vi "downloadBotSpeak.vi"() -> ()   [LabVIEW 2012]
panel:
  out "Current task":string
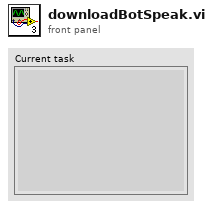
[diagram p1: front panel]
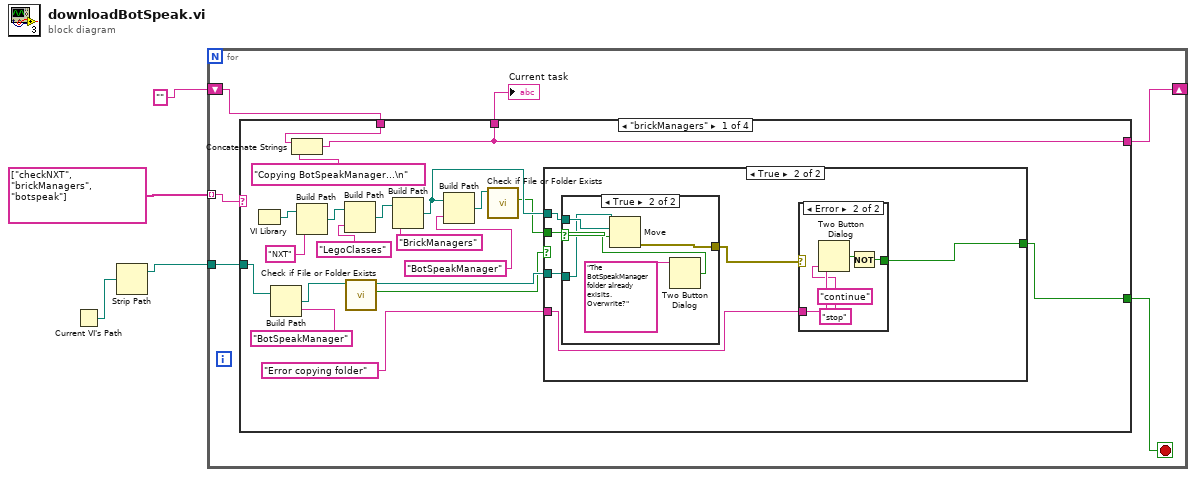
[diagram p0: block diagram]
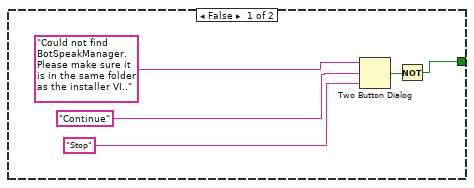
[diagram p2: hidden frame]
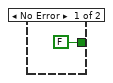
[diagram p3: hidden frame]
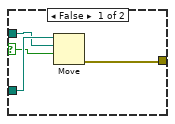
[diagram p4: hidden frame]
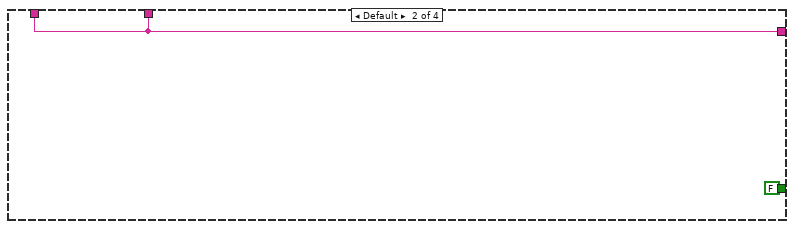
[diagram p5: hidden frame]
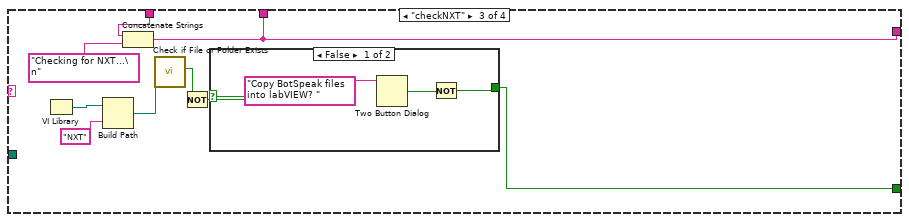
[diagram p6: hidden frame]
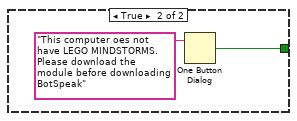
[diagram p7: hidden frame]
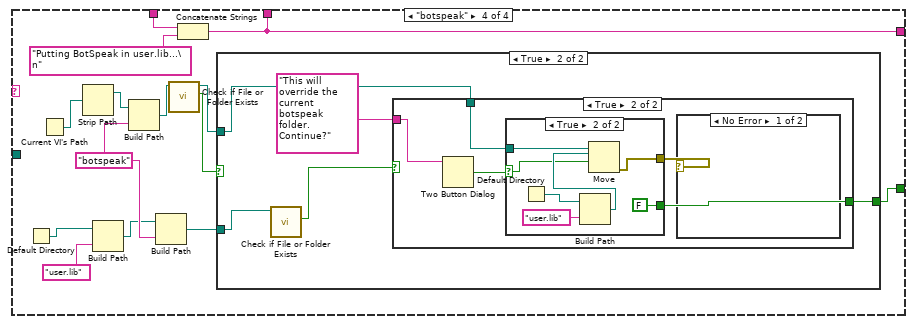
[diagram p8: hidden frame]
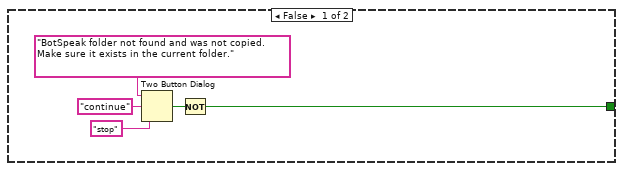
[diagram p9: hidden frame]
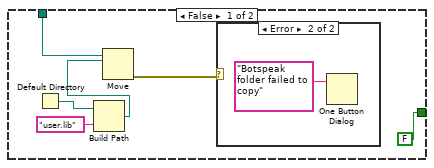
[diagram p10: hidden frame]
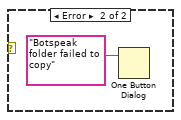
[diagram p12: hidden frame]
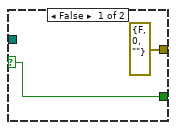
[diagram p13: hidden frame]
diagram:
  n1 = Current VI's Path() -> (path=w3:path)
  n2 = Strip Path(path=w3) -> (stripped path=w2:path)  [unwired: 1 out]
  n3 = for {
    tunnel: string[] ["checkNXT", "brickManagers", "botspeak"] -> [w10] mode=indexing
    tunnel: w2 -> [w9]
    shift-right: [w8] -> _
    shift-left: "" -> [w6]
    stop <- w7 stop-if-true
    n4 = case shown="\"brickManagers\"" w10 {
      tunnel: w9 -> [w25 _ _ _]
      tunnel: w6 -> [w15 w57 w62 w86]
      tunnel: [w11 w57 w59 w73] -> w8
      tunnel: [w12 FALSE ("T button?") w60 w79] -> w7
      tunnel: [w11 w57 w59 w73] -> w5
      frame "brickManagers" {
        n5 = VI Library() -> (path=w30:path)
        n6 = Build Path(base path=w25, name or relative path="BotSpeakManager") -> (appended path=w17:path)
        n7 = Concatenate Strings(w15, "Copying BotSpeakManager...\n" ("string")) -> (w11:string)
        n8 = Build Path(base path=w30, name or relative path="NXT") -> (appended path=w23:path)
        n9 = Build Path(base path=w23, name or relative path="LegoClasses") -> (appended path=w29:path)
        n10 = call <vilib>:"Check if File or Folder Exists.vi"("path"=w17) -> ("file or folder exists?"=w16:bool, "dup path"=w18:path)  [unwired: 8 in, 1 out]
        n11 = Build Path(base path=w29, name or relative path="BrickManagers") -> (appended path=w22:path)
        n12 = Build Path(base path=w22, name or relative path="BotSpeakManager") -> (appended path=w20:path)
        n13 = call <vilib>:"Check if File or Folder Exists.vi"("path"=w20) -> ("file or folder exists?"=w19:bool)  [unwired: 8 in, 2 out]
        n14 = case shown="True" w16 {
          tunnel: w22 -> [_ w41]
          tunnel: w19 -> [_ w40]
          tunnel: w18 -> [_ w39]
          tunnel: "Error copying folder" -> [_ w37]
          tunnel: [w31 w36] -> w12
          frame False {
            n15 = Two Button Dialog(message="Could not find BotSpeakManager. Please make sure it is in the same folder as the installer VI..", 1:"Stop" ("F button name (\"Cancel\")"), 2:"Continue" ("T button name (\"OK\")")) -> (T button?=w32:bool)
            n16 = Not(x=w32) -> (.not. x?=w31:bool)
          }
          frame True {
            n17 = case shown="True" w40 {
              selector: w40 -> [w48 _]
              tunnel: w41 -> [w50 w56]
              tunnel: w39 -> [w51 w55]
              tunnel: [w49 w52] -> w38
              frame False {
                n18 = Move(source path=w51, 9:w48, 10:w50) -> (error out=w49:errorcluster)  [unwired: 2 in, 2 out]
              }
              frame True {
                n19 = Two Button Dialog(message="The BotSpeakManager folder already exisits. Overwrite?") -> (T button?=w54:bool)  [unwired: 2 in]
                n20 = Move(source path=w55, 9:w54, 10:w56) -> (error out=w52:errorcluster)  [unwired: 2 in, 2 out]
              }
            }
            n21 = case shown="Error" w38 {
              tunnel: w37 -> [_ w47]
              tunnel: [FALSE ("T button?") w43] -> w36
              frame No Error {
              }
              frame Error {
                n22 = Two Button Dialog(message=w47, 1:"stop" ("F button name (\"Cancel\")"), 2:"continue" ("T button name (\"OK\")")) -> (T button?=w44:bool)
                n23 = Not(x=w44) -> (.not. x?=w43:bool)
              }
            }
          }
        }
      }
      frame Default {
      }
      frame "checkNXT" {
        n24 = VI Library() -> (path=w67:path)
        n25 = Build Path(base path=w67, name or relative path="NXT") -> (appended path=w65:path)
        n26 = Concatenate Strings(w62, "Checking for NXT...\n" ("string")) -> (w59:string)
        n27 = call <vilib>:"Check if File or Folder Exists.vi"("path"=w65) -> ("file or folder exists?"=w64:bool)  [unwired: 8 in, 2 out]
        n28 = Not(x=w64) -> (.not. x?=w63:bool)
        n29 = case shown="False" w63 {
          tunnel: [w69 w71] -> w60
          frame False {
            n30 = Two Button Dialog(message="Copy BotSpeak files into labVIEW? ") -> (T button?=w70:bool)  [unwired: 2 in]
            n31 = Not(x=w70) -> (.not. x?=w69:bool)
          }
          frame True {
            n32 = One Button Dialog(message="This computer oes not have LEGO MINDSTORMS. Please download the module before downloading BotSpeak") -> (true=w71:bool)  [unwired: 1 in]
          }
        }
      }
      frame "botspeak" {
        w76 = "botspeak" ("name or relative path")
        n33 = Default Directory() -> (w78:path)
        n34 = Current VI's Path() -> (path=w83:path)
        n35 = Strip Path(path=w83) -> (stripped path=w84:path)  [unwired: 1 out]
        n36 = Build Path(base path=w78, name or relative path="user.lib") -> (appended path=w75:path)
        n37 = Build Path(base path=w84, name or relative path=w76) -> (appended path=w82:path)
        n38 = Build Path(base path=w75, name or relative path=w76) -> (appended path=w74:path)
        n39 = call <vilib>:"Check if File or Folder Exists.vi"("path"=w82) -> ("file or folder exists?"=w81:bool, "dup path"=w80:path)  [unwired: 8 in, 1 out]
        n40 = Concatenate Strings(w86, "Putting BotSpeak in user.lib...\n" ("string")) -> (w73:string)
        n41 = case shown="True" w81 {
          tunnel: w80 -> [_ w93]
          tunnel: [w87 w92] -> w79
          tunnel: w74 -> [_ w95]
          frame False {
            n42 = Two Button Dialog(message="BotSpeak folder not found and was not copied. Make sure it exists in the current folder.", 1:"stop" ("F button name (\"Cancel\")"), 2:"continue" ("T button name (\"OK\")")) -> (T button?=w88:bool)
            n43 = Not(x=w88) -> (.not. x?=w87:bool)
          }
          frame True {
            n44 = call <vilib>:"Check if File or Folder Exists.vi"("path"=w95) -> ("file or folder exists?"=w94:bool)  [unwired: 8 in, 2 out]
            n45 = case shown="True" w94 {
              tunnel: "This will override the current botspeak folder. Continue?" ("message") -> [_ w108]
              tunnel: w93 -> [w98 w106]
              tunnel: [FALSE w105] -> w92
              frame False {
                n46 = Default Directory() -> (w101:path)
                n47 = Build Path(base path=w101, name or relative path="user.lib") -> (appended path=w99:path)
                n48 = Move(source path=w98, 10:w99) -> (error out=w97:errorcluster)  [unwired: 3 in, 2 out]
                n49 = case shown="Error" w97 {
                  frame No Error {
                  }
                  frame Error {
                    n50 = One Button Dialog(message="Botspeak folder failed to copy") -> ()  [unwired: 1 in, 1 out]
                  }
                }
              }
              frame True {
                n51 = Two Button Dialog(message=w108) -> (T button?=w107:bool)  [unwired: 2 in]
                n52 = case shown="True" w107 {
                  selector: w107 -> [w111 w114]
                  tunnel: w106 -> [_ w118]
                  tunnel: [w111 FALSE] -> w105
                  tunnel: [errorcluster {"status"=FALSE, "code"=0, "source"=""} ("error out") w112] -> w104
                  frame False {
                  }
                  frame True {
                    n53 = Default Directory() -> (w117:path)
                    n54 = Build Path(base path=w117, name or relative path="user.lib") -> (appended path=w115:path)
                    n55 = Move(source path=w118, 9:w114, 10:w115) -> (error out=w112:errorcluster)  [unwired: 2 in, 2 out]
                  }
                }
                n56 = case shown="No Error" w104 {
                  frame No Error {
                  }
                  frame Error {
                    n57 = One Button Dialog(message="Botspeak folder failed to copy") -> ()  [unwired: 1 in, 1 out]
                  }
                }
              }
            }
          }
        }
      }
    }
    "Current task" <- w5
  }
